vi "RobotPositionReplacementTestPasse.vi"(6 "Atacando contra?":bool, 7 "id":i32, 8 "IA State Input":T1, 9 "Position Ball":dbl[](array[numeric])) -> (2 "Position Robot":dbl[](array[numeric]))   [LabVIEW 2017]
uses:
  Core/AI Input.ctl
  Core/AI Robot.ctl
  Intel/Functions Enum.ctl
  Intel/AttackerStates.ctl
  Path Planning/RRT/PathDests.ctl
  Path Planning/RRT/PathDest.ctl
  Core/AI Ball.ctl
  Core/Field Size.ctl
  Core/AI Judge.ctl
  Intel/Command Enum.ctl
  Util/Events/Events.ctl
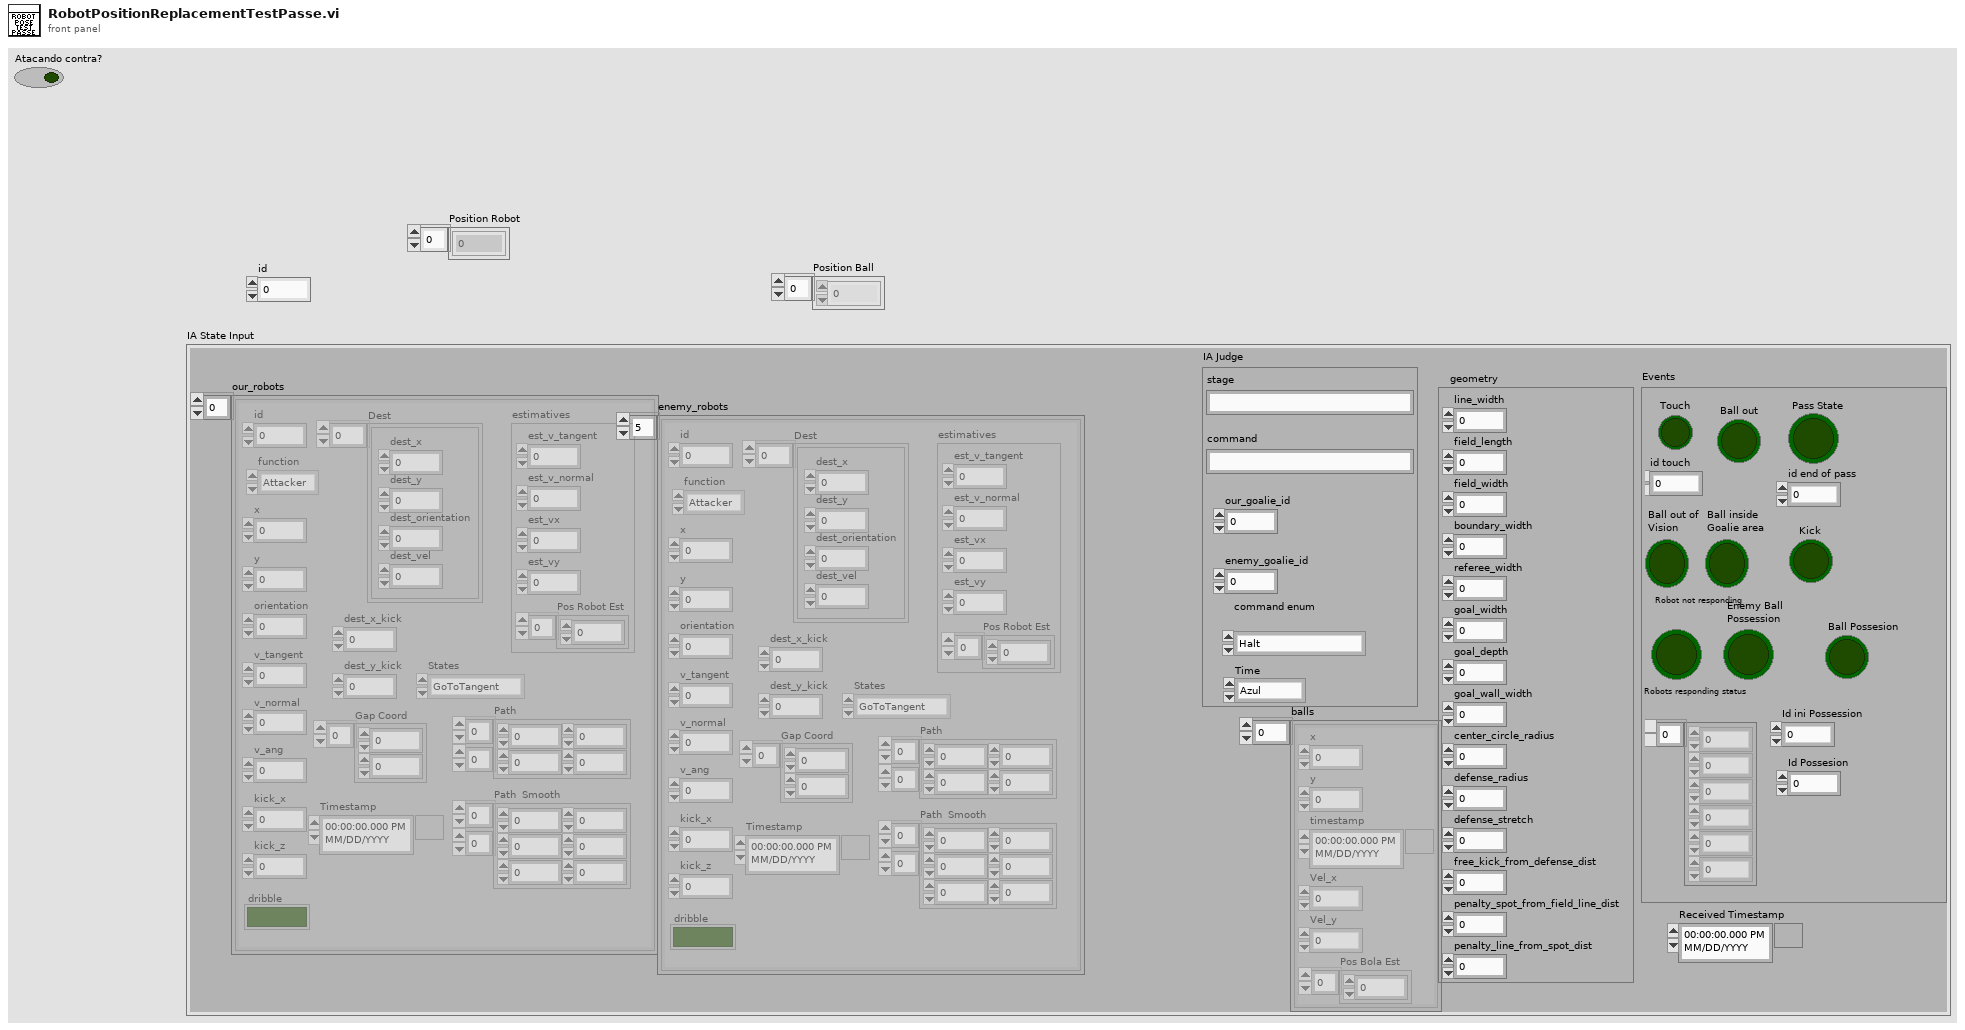
[diagram p1: front panel]
types:
  T1 = typedef "AI Input.ctl" = cluster{"our_robots":T2[], "enemy_robots":T2[], "balls":T7[], "geometry":T8, "IA Judge":T9, "Received Timestamp":timestamp, "Events":T11}
  T2 = typedef "AI Robot.ctl" = cluster{"id":u32, "function":T3, "x":dbl, "y":dbl, "orientation":dbl, "v_tangent":dbl, "v_normal":dbl, "v_ang":dbl, "kick_x":dbl, "kick_z":dbl, "dribble":bool, "Timestamp":timestamp, "estimatives":cluster{"est_v_tangent":dbl, "est_v_normal":dbl, "est_vx":dbl, "est_vy":dbl, "Pos Robot Est":dbl[]}, "dest_x_kick":dbl, "dest_y_kick":dbl, "Gap Coord":dbl[], "States":T4, "Path ":dbl[][], "Path  Smooth":dbl[][], "Dest":T5}
  T3 = typedef "Functions Enum.ctl" = enum16{"Attacker", "Goalie", "Defender", "Striker", "Goto 0", "Dummy", "Kicker", "ZigZag"}
  T4 = typedef "AttackerStates.ctl" = enum16{"Pass", "GoToTangent", "BallGetting", "GoToKick", ""}
  T5 = typedef "PathDests.ctl" = T6[]
  T6 = typedef "PathDest.ctl" = cluster{"dest_x":dbl, "dest_y":dbl, "dest_orientation":dbl, "dest_vel":dbl}
  T7 = typedef "AI Ball.ctl" = cluster{"x":dbl, "y":dbl, "timestamp":timestamp, "Vel_x":dbl, "Vel_y":dbl, "Pos Bola Est":dbl[]}
  T8 = typedef "Field Size.ctl" = cluster{"line_width":u32, "field_length":u32, "field_width":u32, "boundary_width":u32, "referee_width":u32, "goal_width":u32, "goal_depth":u32, "goal_wall_width":u32, "center_circle_radius":u32, "defense_radius":u32, "defense_stretch":u32, "free_kick_from_defense_dist":u32, "penalty_spot_from_field_line_dist":u32, "penalty_line_from_spot_dist":u32}
  T9 = typedef "AI Judge.ctl" = cluster{"stage":string, "command":string, "our_goalie_id":dbl, "enemy_goalie_id":dbl, "command enum":T10, "Time":enum16{"Azul", "Amarelo"}}
  T10 = typedef "Command Enum.ctl" = enum16{"Halt", "Stop", "Force Start", "PKA Normal Start", "Prepare Kickoff Ally", "PKE Normal Start", "Prepare Kickoff Enemy", "Prepare Penalty Ally", "PPA Normal Start", "Prepare Penalty Enemy", "PPE Normal Start", "Direct Free Enemy", "Direct Free Ally", "Indirect Free Enemy", "Indirect Free Ally", "Timeout Enemy", "Timeout Ally", "Goal Enemy", "Goal Ally", "Ball Placement Enemy", "Ball Placement Ally", "Normal Half Time", "Extra Time Break", "Extra Half Time", "None", "Post Game"}
  T11 = typedef "Events.ctl" = cluster{"Touch":bool, "Ball out":bool, "id touch":dbl, "Ball out of \nVision":bool, "Ball inside \nGoalie area":bool, "Robot not responding":bool, "Robots responding status":dbl[], "Enemy Ball \nPossession":bool, "Pass State":bool, "id end of pass":dbl, "Kick":bool, "Id ini Possession":dbl, "Ball Possesion":bool, "Id Possesion":dbl}
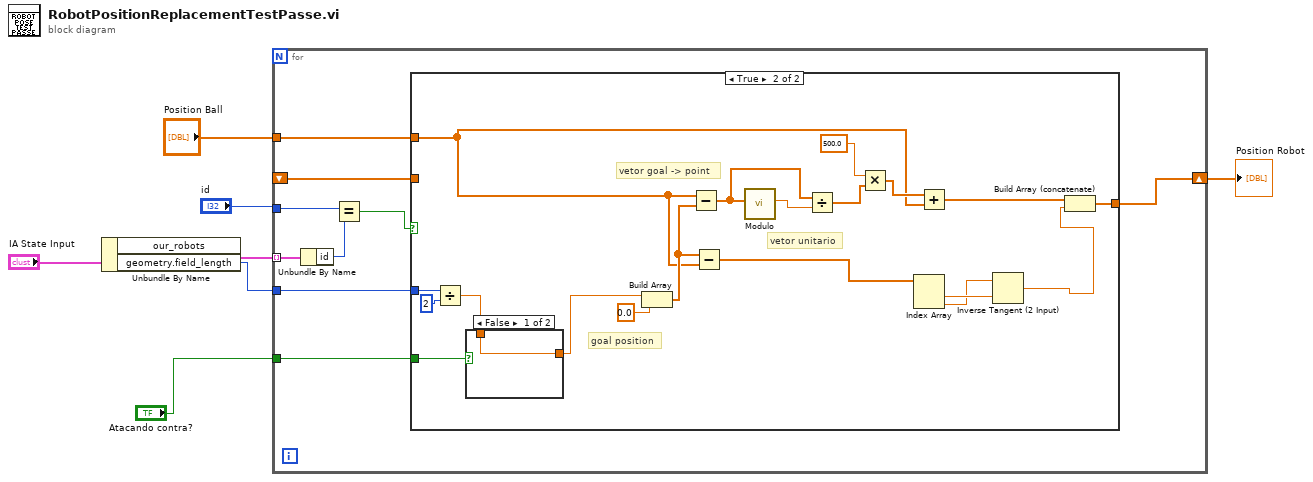
[diagram p0: block diagram]
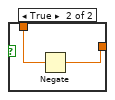
[diagram p3: hidden frame]
diagram:
  n1 = Unbundle By Name("IA State Input") -> ("our_robots"=w6:T2[], "geometry.field_length"=w3:u32)
  n2 = for {
    tunnel: w6 -> [w13] mode=indexing
    tunnel: "id" -> [w16]
    tunnel: "Position Ball" -> [w14]
    tunnel: w3 -> [w11]
    shift-right: [w10] -> w2
    shift-left: _ -> [w9]
    tunnel: "Atacando contra?" -> [w8]
    n3 = Unbundle By Name(w13) -> ("id"=w12:u32)
    n4 = Equal?(x=w16, y=w12) -> (x = y?=w15:bool)
    n5 = case shown="True" w15 {
      tunnel: w14 -> [_ w23]
      tunnel: w11 -> [_ w36]
      tunnel: [w17 w28] -> w10
      tunnel: w9 -> [w17 _]
      tunnel: w8 -> [_ w20]
      frame False {
      }
      frame True {
        # "vetor unitario"
        # "vetor goal -> point"
        # "goal position"
        n6 = Divide(x=w36, y=u32 2) -> (x/y=w19:dbl)
        n7 = case shown="False" w20 {
          tunnel: w19 -> [w37 w39]
          tunnel: [w37 w38] -> w18
          frame False {
          }
          frame True {
            n8 = Negate(x=w39) -> (-x=w38:dbl)
          }
        }
        n9 = Build Array(w18, 0.0 ("element")) -> (w24:dbl[])
        n10 = Subtract(x=w23, y=w24) -> (x-y=w33:dbl[])
        n11 = Subtract(x=w24, y=w23) -> (x-y=w21:dbl[])
        n12 = call "Modulo.vi"("2D vector"=w33) -> ("Modulo"=w32:dbl)  [unwired: 10 in]
        n13 = Divide(x=w33, y=w32) -> (x/y=w22:dbl[])
        n14 = Multiply(x=500.0, y=w22) -> (x*y=w30:dbl[])
        n15 = Index Array(array=w21) -> (element #1=w27:dbl, element #2=w26:dbl)  [unwired: 2 in]
        n16 = Add(x=w30, y=w23) -> (x+y=w29:dbl[])
        n17 = Inverse Tangent (2 Input)(1:w27, 2:w26) -> (0:w25:dbl)
        n18 = Build Array (concatenate)(w29, w25) -> (w28:dbl[])
      }
    }
  }
  "Position Robot" <- w2
